vi "Voice_Check.vi"(8 "error in (no error)":errorcluster, 11 "IN":T1={"step name 1"="", "updata 2"="750~0.22", "limitdata 3"="650~0.101", "load vi name 4"="", "parameter 5"=""}) -> (0 "error out":errorcluster, 3 "Cluster":T2)   [LabVIEW 2013]
uses:
  <vilib>/sound2/lvsound2.llb/Sampling Mode.ctl
  <vilib>/sound2/lvsound2.llb/Sound Data Format.ctl
  <vilib>/measure/matone.llb/Extract Single Tone Information N Chan.vi
  <vilib>/sound2/lvsound2.llb/Sound Input Read (DBL).vi
  <vilib>/measure/NI_MAPro.lvlib
panel:
  out "Array":bool[](array[boolean])
  out "pass":bool
  out "data":waveform(dbl)[](array[waveform])
  # "Hi: 750~0.22"
  # "Lo: 650~0.101"
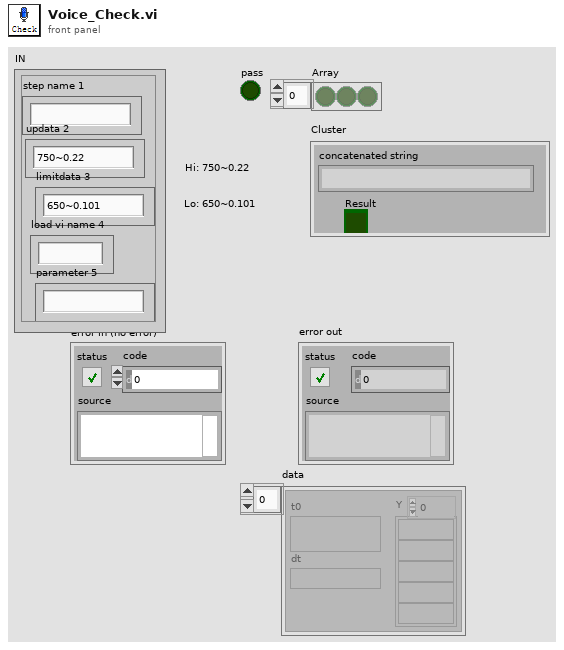
[diagram p1: front panel]
types:
  T1 = cluster{"step name 1":string, "updata 2":string, "limitdata 3":string, "load vi name 4":string, "parameter 5":string}
  T2 = cluster{"concatenated string":string, "Result":bool}
  T3 = typedef "Sound Data Format.ctl" = cluster{"sample rate (S/s)":dbl, "number of channels":i32, "bits per sample":i32}
  T4 = typedef "Sampling Mode.ctl" = i32
  T5 = typedef "Sound Input Task ID.ctl" = u32
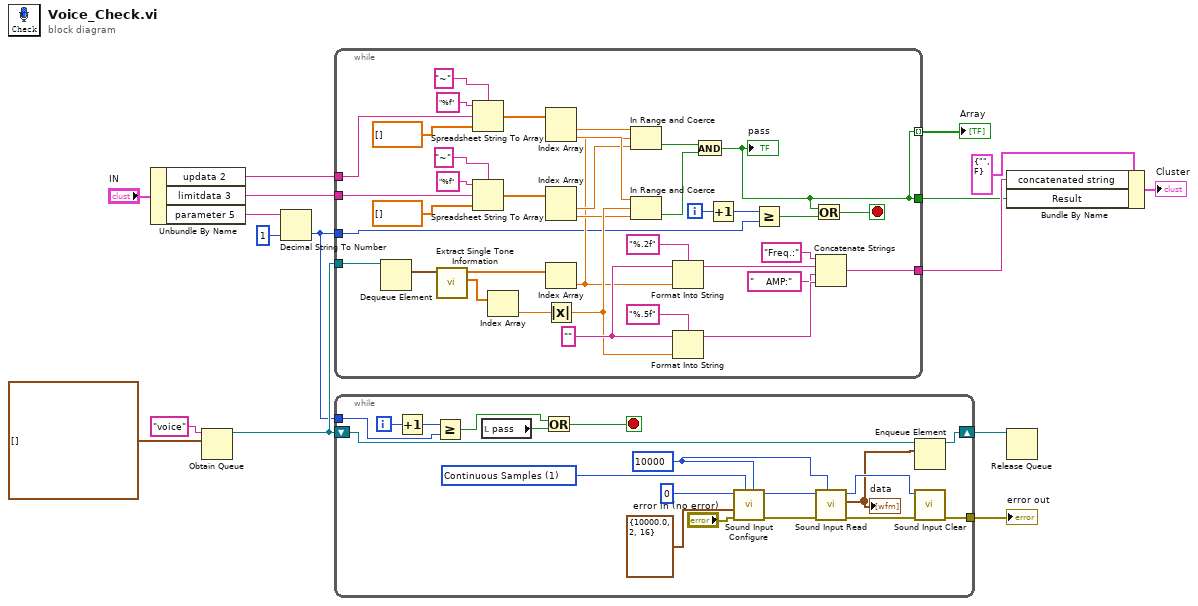
[diagram p0: block diagram]
diagram:
  n1 = Unbundle By Name("IN") -> ("updata 2"=w11:string, "limitdata 3"=w10:string, "parameter 5"=w9:string)
  n2 = Obtain Queue(name (unnamed)="voice", element data type=waveform(dbl)[] [] ("data 2")) -> (queue out=w4:refnum<queue>)  [unwired: 3 in, 2 out]
  n3 = Decimal String To Number(string=w9, default (0L)=1 ("default (0 I32)")) -> (number=w3:i32)  [unwired: 1 in, 1 out]
  n4 = while {
    tunnel: [w43] -> w14
    tunnel: [w19] -> w13
    tunnel: w11 -> [w30]
    tunnel: w10 -> [w29]
    tunnel: w4 -> [w28]
    tunnel: w3 -> [w20]
    tunnel: [w19] -> w1 mode=indexing
    i -> [w18]
    stop <- w22 stop-if-true
    w53 = "" ("initial string")
    n5 = Dequeue Element(queue=w28) -> (element=w27:waveform(dbl)[])  [unwired: 2 in, 3 out]
    n6 = call-poly <vilib>:"Extract Single Tone Information.vi"("time signals in"=w27) -> ("detected amplitudes"=w25:dbl[], "detected frequencies"=w26:dbl[])  [unwired: 3 in, 6 out]
    n7 = Spreadsheet String To Array(delimiter (Tab)="~", format string="%f", spreadsheet string=w30, array type (2D Dbl)=dbl[] []) -> (array=w36:dbl[])
    n8 = Spreadsheet String To Array(delimiter (Tab)="~", format string="%f", spreadsheet string=w29, array type (2D Dbl)=dbl[] []) -> (array=w33:dbl[])
    n9 = Index Array(array=w25) -> (element=w24:dbl)  [unwired: 1 in]
    n10 = Index Array(array=w36) -> (element #1=w35:dbl, element #2=w34:dbl)  [unwired: 2 in]
    n11 = Index Array(array=w33) -> (element #1=w32:dbl, element #2=w31:dbl)  [unwired: 2 in]
    n12 = Index Array(array=w26) -> (element=w23:dbl)  [unwired: 1 in]
    n13 = Absolute Value(x=w24) -> (abs(x)=w46:dbl)
    n14 = In Range and Coerce(upper limit=w35, x=w23, lower limit=w32) -> (In Range?=w45:bool)  [unwired: 1 out]
    n15 = In Range and Coerce(upper limit=w34, x=w46, lower limit=w31) -> (In Range?=w44:bool)  [unwired: 1 out]
    n16 = Format Into String(format string="%.2f", initial string=w53, w23) -> (resulting string=w51:string)  [unwired: 1 in, 1 out]
    n17 = Format Into String(format string="%.5f", initial string=w53, w46) -> (resulting string=w49:string)  [unwired: 1 in, 1 out]
    n18 = And(x=w45, y=w44) -> (x .and. y?=w19:bool)
    "pass" <- w19
    n19 = Increment(x=w18) -> (x+1=w17:i32)
    n20 = Greater Or Equal?(x=w17, y=w20) -> (x >= y?=w21:bool)
    n21 = Or(x=w19, y=w21) -> (x .or. y?=w22:bool)
    n22 = Concatenate Strings("Freq.:" ("string"), w51, "    AMP:" ("string"), w49) -> (w43:string)
  }
  "Array" <- w1
  n23 = while {
    tunnel: w3 -> [w60]
    shift-right: [w61] -> w5
    shift-left: w4 -> [w62]
    tunnel: [w56] -> w2
    i -> [w55]
    stop <- w59 stop-if-true
    w71 = 10000 ("Number of Samples/ch")
    w70 = T4 1 items=["Finite Samples", "Continuous Samples"] ("sample mode")
    n24 = Increment(x=w55) -> (x+1=w54:i32)
    n25 = Greater Or Equal?(x=w54, y=w60) -> (x >= y?=w58:bool)
    n26 = local read "pass"() -> (w57:bool)
    n27 = Or(x=w58, y=w57) -> (x .or. y?=w59:bool)
    n28 = call <vilib>:"Sound Input Configure.vi"("number of samples/ch"=w71, "sample mode"=w70, "error in (no error)"="error in (no error)", "sound format"=T3 {"sample rate (S/s)"=10000.0, "number of channels"=2, "bits per sample"=16} ("Sound Format"), "device ID"=u32 0 ("Device ID")) -> ("error out"=w65:errorcluster, "task ID"=w67:T5)  [unwired: 2 in, 3 out]
    n29 = call-poly <vilib>:"Sound Input Read.vi"("number of samples/ch"=w71, "error in (no error)"=w65, "task ID"=w67) -> ("error out"=w69:errorcluster, "data"=w63:waveform(dbl)[], "task ID out"=w68:T5)  [unwired: 1 in, 5 out]
    "data" <- w63
    n30 = Enqueue Element(queue=w62, element=w63) -> (queue out=w61:refnum<queue>)  [unwired: 2 in, 2 out]
    n31 = call <vilib>:"Sound Input Clear.vi"("error in (no error)"=w69, "task ID"=w68) -> ("error out"=w56:errorcluster)  [unwired: 9 out]
  }
  "error out" <- w2
  n32 = Bundle By Name(cluster=T2 {"concatenated string"="", "Result"=FALSE} ("Cluster"), "concatenated string"=w14, "Result"=w13) -> (→"Cluster":T2)
  n33 = Release Queue(queue=w5) -> ()  [unwired: 2 in, 3 out]
